vi "Configure Multi Eval Meas Limit Equalizer Spectrum Flatness.vi"(0 "VISA resource name":refnum<visa-resource-name>, 1 "Range 1 (0.0)":dbl format="%^.3e", 2 "Max 1 Min 2 (0.0)":dbl format="%^.3e", 3 "Edge Frequency (0Hz)":dbl format="%#.9p", 5 "Instance (1)":T1=1, 7 "Modulation (Pi/2-BPSK)":i32(ring) items=["Pi/2-BPSK", "Pi/2-BPSK With Shaping", "QPSK", "16-QAM", "64-QAM", "256-QAM"], 9 "Enabled (Off)":bool, 11 "error in (no error)":errorcluster, 12 "Range 2 (0.0)":dbl format="%^.3e", 13 "Max 2 Min 1 (0.0)":dbl format="%^.3e") -> (4 "VISA resource name out":refnum<visa-resource-name>, 15 "error out":errorcluster)   [LabVIEW 2020, in "Rohde&Schwarz CMWXP NR FR1 Measurement.lvlib"]
doc: "Defines limits for the equalizer spectrum flatness.\n\nAttributes:\nRSCMWXPNRFR1M_ATTR_MULTI_EVAL_MEAS_LIMIT_PI_2_EQUALIZER_SPECTRUM_FLATNESS\nRSCMWXPNRFR1M_ATTR_MULTI_EVAL_MEAS_LIMIT_BPSK_SHAPING_EQUALIZER_SPECTRUM_FLATNESS\nRSCMWXPNRFR1M_ATTR_MULTI_EVAL_MEAS_LIMIT_QPSK_EQUALIZER_SPECTRUM_FLATNESS\nRSCMWXPNRFR1M_ATTR_MULTI_EVAL_MEAS_LIMIT_QAM_EQUALIZER_SPECTRUM_FLATNESS\n\nRemote-control commands:\nCONFigure:NRSub:MEAS<i>:MEValuation:LIMit:PHBPsk:ESFLatness\nCONFigure:NRSub:MEAS<i>:MEValuation:LIMit:BPWShaping:ESFLatness\nCONFigure:NRSub:MEAS<i>:MEValuation:LIMit:QPSK:ESFLatness\nCONFigure:NRSub:MEAS<i>:MEValuation:LIMit:QAM<order>:ESFLatness"
uses:
  <instrlib>/Rohde&Schwarz CMWXP NR FR1 Measurement/Rohde&Schwarz CMWXP NR FR1 Measurement.lvlib
  <instrlib>/Rohde&Schwarz CMWXP NR FR1 Measurement/Private/_Instance.ctl
  <instrlib>/Rohde&Schwarz CMWXP NR FR1 Measurement/Private/rsidr_core.llb/rsidr_core.lvlib
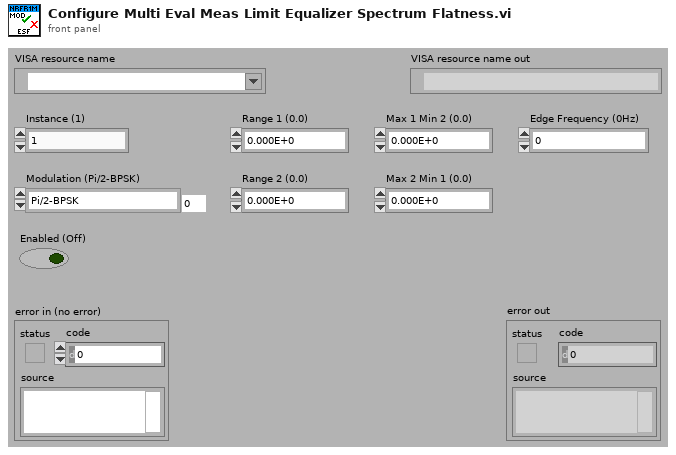
[diagram p1: front panel]
types:
  T1 = typedef "Rohde&Schwarz CMWXP NR FR1 Measurement.lvlib/_Instance.ctl" = i32
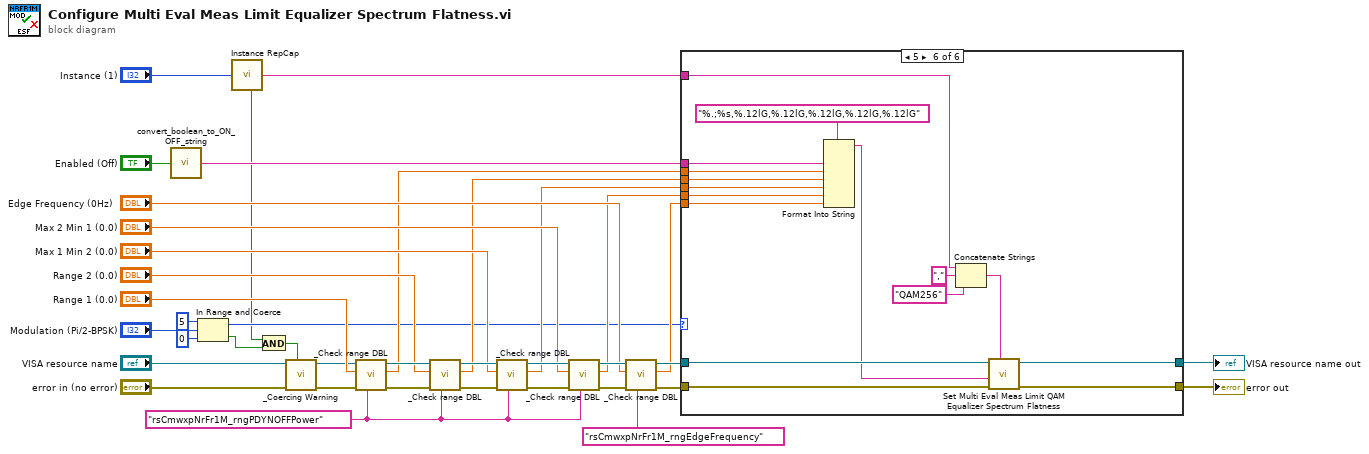
[diagram p0: block diagram]
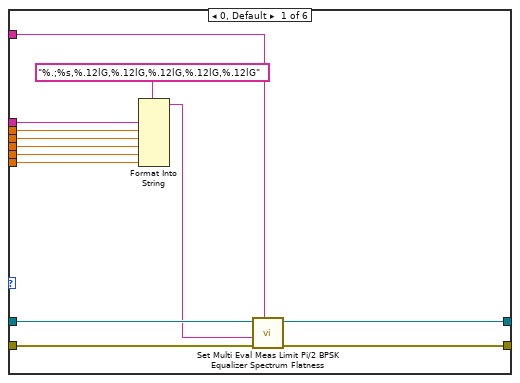
[diagram p2: hidden frame]
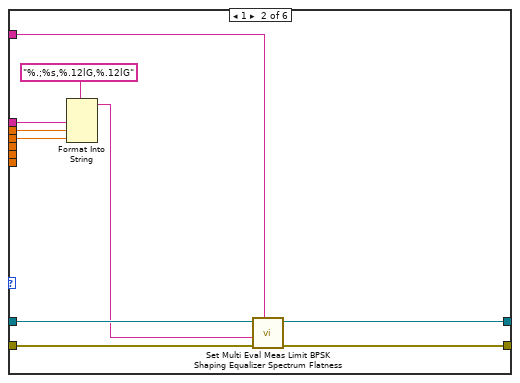
[diagram p3: hidden frame]
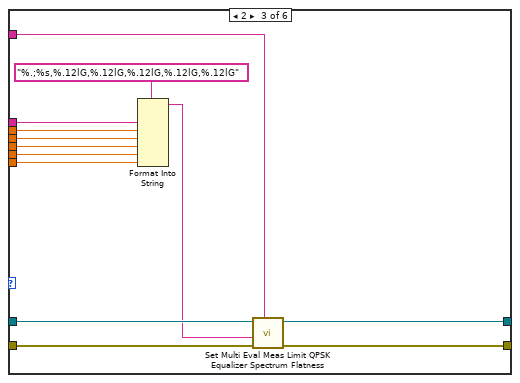
[diagram p4: hidden frame]
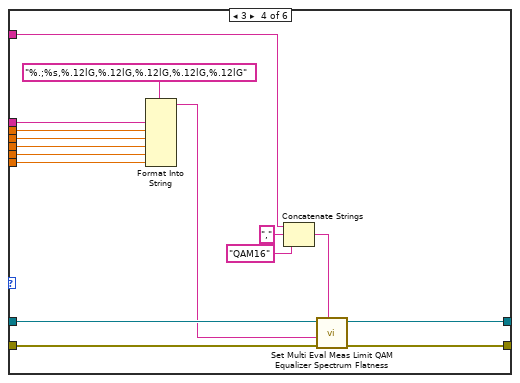
[diagram p5: hidden frame]
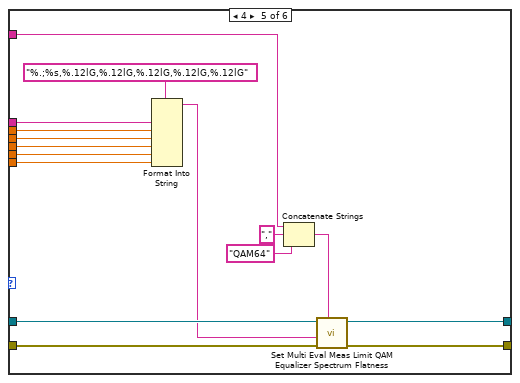
[diagram p6: hidden frame]
diagram:
  w19 = "rsCmwxpNrFr1M_rngPDYNOFFPower" ("Range Table Identifier")
  n1 = call <instrlib>:"convert_boolean_to_ON_OFF_string.vi"("boolean value in"="Enabled (Off)") -> ("string value out"=w12:string)  [unwired: 4 in]
  n2 = In Range and Coerce(upper limit=5, x="Modulation (Pi/2-BPSK)", lower limit=0) -> (coerced(x)=w11:i32, In Range?=w1:bool)
  n3 = call <instrlib>:"Instance RepCap.vi"("Instance In"="Instance (1)") -> ("In Range?"=w7:bool, "RepCap Identifier Out"=w38:string)  [unwired: 1 in]
  n4 = And(x=w7, y=w1) -> (x .and. y?=w2:bool)
  n5 = call <instrlib>:"_Coercing Warning.vi"("In Range?"=w2, "error in (no error)"="error in (no error)", "VISA resource name"="VISA resource name") -> ("error out"=w4:errorcluster, "VISA resource name out"=w3:refnum<visa-resource-name>)  [unwired: 7 in]
  n6 = call <instrlib>:"_Check range DBL.vi"("Range Table Identifier"=w19, "error in (no error)"=w4, "DBL Value In"="Range 1 (0.0)", "VISA resource name"=w3) -> ("error out"=w36:errorcluster, "DBL Value Out"=w13:dbl, "VISA resource name out"=w35:refnum<visa-resource-name>)  [unwired: 5 in]
  n7 = call <instrlib>:"_Check range DBL.vi"("Range Table Identifier"=w19, "error in (no error)"=w36, "DBL Value In"="Range 2 (0.0)", "VISA resource name"=w35) -> ("error out"=w34:errorcluster, "DBL Value Out"=w14:dbl, "VISA resource name out"=w33:refnum<visa-resource-name>)  [unwired: 5 in]
  n8 = call <instrlib>:"_Check range DBL.vi"("Range Table Identifier"=w19, "error in (no error)"=w34, "DBL Value In"="Max 1 Min 2 (0.0)", "VISA resource name"=w33) -> ("error out"=w32:errorcluster, "DBL Value Out"=w15:dbl, "VISA resource name out"=w31:refnum<visa-resource-name>)  [unwired: 5 in]
  n9 = call <instrlib>:"_Check range DBL.vi"("Range Table Identifier"=w19, "error in (no error)"=w32, "DBL Value In"="Max 2 Min 1 (0.0)", "VISA resource name"=w31) -> ("error out"=w30:errorcluster, "DBL Value Out"=w16:dbl, "VISA resource name out"=w29:refnum<visa-resource-name>)  [unwired: 5 in]
  n10 = call <instrlib>:"_Check range DBL.vi"("Range Table Identifier"="rsCmwxpNrFr1M_rngEdgeFrequency", "error in (no error)"=w30, "DBL Value In"="Edge Frequency (0Hz)", "VISA resource name"=w29) -> ("error out"=w27:errorcluster, "DBL Value Out"=w17:dbl, "VISA resource name out"=w28:refnum<visa-resource-name>)  [unwired: 5 in]
  n11 = case shown="5" w11 {
    tunnel: [w52 w62 w75 w91 w107 w123] -> w20
    tunnel: [w51 w61 w74 w90 w106 w122] -> w21
    tunnel: w38 -> [w50 w60 w73 w87 w103 w119]
    tunnel: w28 -> [w49 w59 w72 w89 w105 w121]
    tunnel: w27 -> [w48 w58 w71 w88 w104 w120]
    tunnel: w17 -> [w40 _ w63 w76 w92 w114]
    tunnel: w16 -> [w41 _ w64 w77 w93 w113]
    tunnel: w15 -> [w42 _ w65 w78 w94 w112]
    tunnel: w14 -> [w43 w53 w66 w79 w95 w111]
    tunnel: w13 -> [w44 w54 w67 w80 w96 w110]
    tunnel: w12 -> [w45 w55 w68 w81 w97 w109]
    frame 0, Default {
      n12 = Format Into String(format string="%.;%s,%.12lG,%.12lG,%.12lG,%.12lG,%.12lG", w45, w44, w43, w42, w41, w40) -> (resulting string=w46:string)  [unwired: 2 in, 1 out]
      n13 = call "Set Multi Eval Meas Limit Pi/2 BPSK Equalizer Spectrum Flatness"("Repeated Capabilities"=w50, "error in (no error)"=w48, "Multi Eval Meas Limit Pi/2 BPSK Equalizer Spectrum Flatness ()"=w46, "instrument handle"=w49) -> ("error out"=w52:errorcluster, "instrument handle out"=w51:refnum<visa-resource-name>)  [unwired: 6 in]
    }
    frame 1 {
      n14 = Format Into String(format string="%.;%s,%.12lG,%.12lG", w55, w54, w53) -> (resulting string=w56:string)  [unwired: 2 in, 1 out]
      n15 = call "Set Multi Eval Meas Limit BPSK Shaping Equalizer Spectrum Flatness"("Repeated Capabilities"=w60, "error in (no error)"=w58, "Multi Eval Meas Limit BPSK Shaping Equalizer Spectrum Flatness ()"=w56, "instrument handle"=w59) -> ("error out"=w62:errorcluster, "instrument handle out"=w61:refnum<visa-resource-name>)  [unwired: 6 in]
    }
    frame 2 {
      n16 = Format Into String(format string="%.;%s,%.12lG,%.12lG,%.12lG,%.12lG,%.12lG", w68, w67, w66, w65, w64, w63) -> (resulting string=w69:string)  [unwired: 2 in, 1 out]
      n17 = call "Set Multi Eval Meas Limit QPSK Equalizer Spectrum Flatness"("Repeated Capabilities"=w73, "error in (no error)"=w71, "Multi Eval Meas Limit QPSK Equalizer Spectrum Flatness ()"=w69, "instrument handle"=w72) -> ("error out"=w75:errorcluster, "instrument handle out"=w74:refnum<visa-resource-name>)  [unwired: 6 in]
    }
    frame 3 {
      n18 = Format Into String(format string="%.;%s,%.12lG,%.12lG,%.12lG,%.12lG,%.12lG", w81, w80, w79, w78, w77, w76) -> (resulting string=w82:string)  [unwired: 2 in, 1 out]
      n19 = Concatenate Strings(w87, "," ("string"), "QAM16" ("string")) -> (w84:string)
      n20 = call "Set Multi Eval Meas Limit QAM Equalizer Spectrum Flatness"("Repeated Capabilities"=w84, "error in (no error)"=w88, "Multi Eval Meas Limit QAM Equalizer Spectrum Flatness ()"=w82, "instrument handle"=w89) -> ("error out"=w91:errorcluster, "instrument handle out"=w90:refnum<visa-resource-name>)  [unwired: 6 in]
    }
    frame 4 {
      n21 = Format Into String(format string="%.;%s,%.12lG,%.12lG,%.12lG,%.12lG,%.12lG", w97, w96, w95, w94, w93, w92) -> (resulting string=w98:string)  [unwired: 2 in, 1 out]
      n22 = Concatenate Strings(w103, "," ("string"), "QAM64" ("string")) -> (w100:string)
      n23 = call "Set Multi Eval Meas Limit QAM Equalizer Spectrum Flatness"("Repeated Capabilities"=w100, "error in (no error)"=w104, "Multi Eval Meas Limit QAM Equalizer Spectrum Flatness ()"=w98, "instrument handle"=w105) -> ("error out"=w107:errorcluster, "instrument handle out"=w106:refnum<visa-resource-name>)  [unwired: 6 in]
    }
    frame 5 {
      n24 = Format Into String(format string="%.;%s,%.12lG,%.12lG,%.12lG,%.12lG,%.12lG", w109, w110, w111, w112, w113, w114) -> (resulting string=w115:string)  [unwired: 2 in, 1 out]
      n25 = Concatenate Strings(w119, "," ("string"), "QAM256" ("string")) -> (w116:string)
      n26 = call "Set Multi Eval Meas Limit QAM Equalizer Spectrum Flatness"("Repeated Capabilities"=w116, "error in (no error)"=w120, "Multi Eval Meas Limit QAM Equalizer Spectrum Flatness ()"=w115, "instrument handle"=w121) -> ("error out"=w123:errorcluster, "instrument handle out"=w122:refnum<visa-resource-name>)  [unwired: 6 in]
    }
  }
  "error out" <- w20
  "VISA resource name out" <- w21
